vi "ZM_State_heating.vi"(6 "T":u32[](array[numeric])=[300, 180000, 300, 5000, 180000, 3000], 9 "ZB":bool[](array[boolean])=[FALSE, FALSE], 10 "XB":bool[](array[boolean])=[FALSE, FALSE, FALSE, FALSE, FALSE], 11 "Z_In":T4={"Z_Source"=enum."local disabled", "Z_State"=enum."alarm", "ZM_State"=enum."initialization"}) -> (1 "t":u32, 3 "Z_Out":T4={"Z_Source"=enum."local disabled", "Z_State"=enum."alarm", "ZM_State"=enum."initialization"}, 4 "ZM_State_next":u32)   [LabVIEW 2019, in "Heating.lvlib"]
uses:
  Heating.lvlib
  ctl/Y_source.ctl
  ctl/Z_State.ctl
  ctl/ZM_State.ctl
  Trigers/RS.vi
  Timer Delay/Timer.vi
  Userlib.lvlib
panel:
  out "End":bool
  out "Stop":bool
  out "Start":bool
  # "Ki_XB01 contactor on"
  # "Ki_XB02 contactor off"
  # "XB24 local hand on"
  # "heating end"
  # "cooling end"
  # "Ki_ZB01 contactor on reg"
  # "Ki_ZB02 contactor off reg"
  # "T_start_delay"
  # "T_heat_start"
  # "T_stop_delay"
  # "T_set_min"
  # "T_heat_stop"
  # "T_restart_delay"
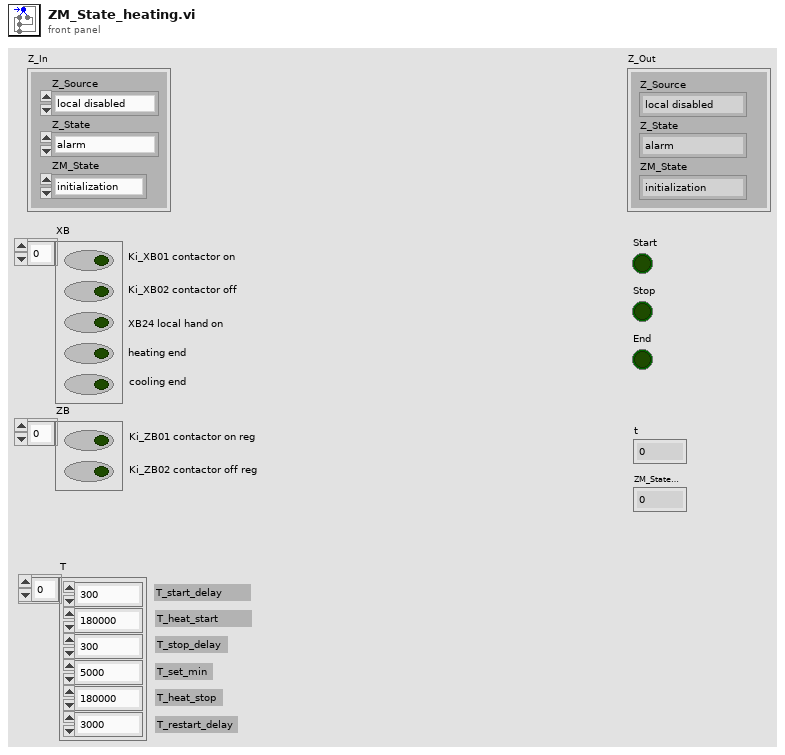
[diagram p1: front panel]
types:
  T1 = typedef "Heating.lvlib/Y_source.ctl" = enum8{"initialize", "local disabled", "local hand", "hand", "auto", "dist"}
  T2 = typedef "Heating.lvlib/Z_State.ctl" = enum8{"initialization", "alarm", "disabled", "not ready", "stop ready", "reserv", "switched off", "reserv2", "switched on", "check", "on min", "decrease out", "on", "increase out", "on max"}
  T3 = typedef "Heating.lvlib/ZM_State.ctl" = enum8{"initialization", "stop", "start_cmd", "contactor_on_cmd", "heating", "on", "stop_cmd", "power_down", "contactor_off_cmd", "cooling", "restart_delay"}
  T4 = cluster{"Z_Source":T1, "Z_State":T2, "ZM_State":T3}
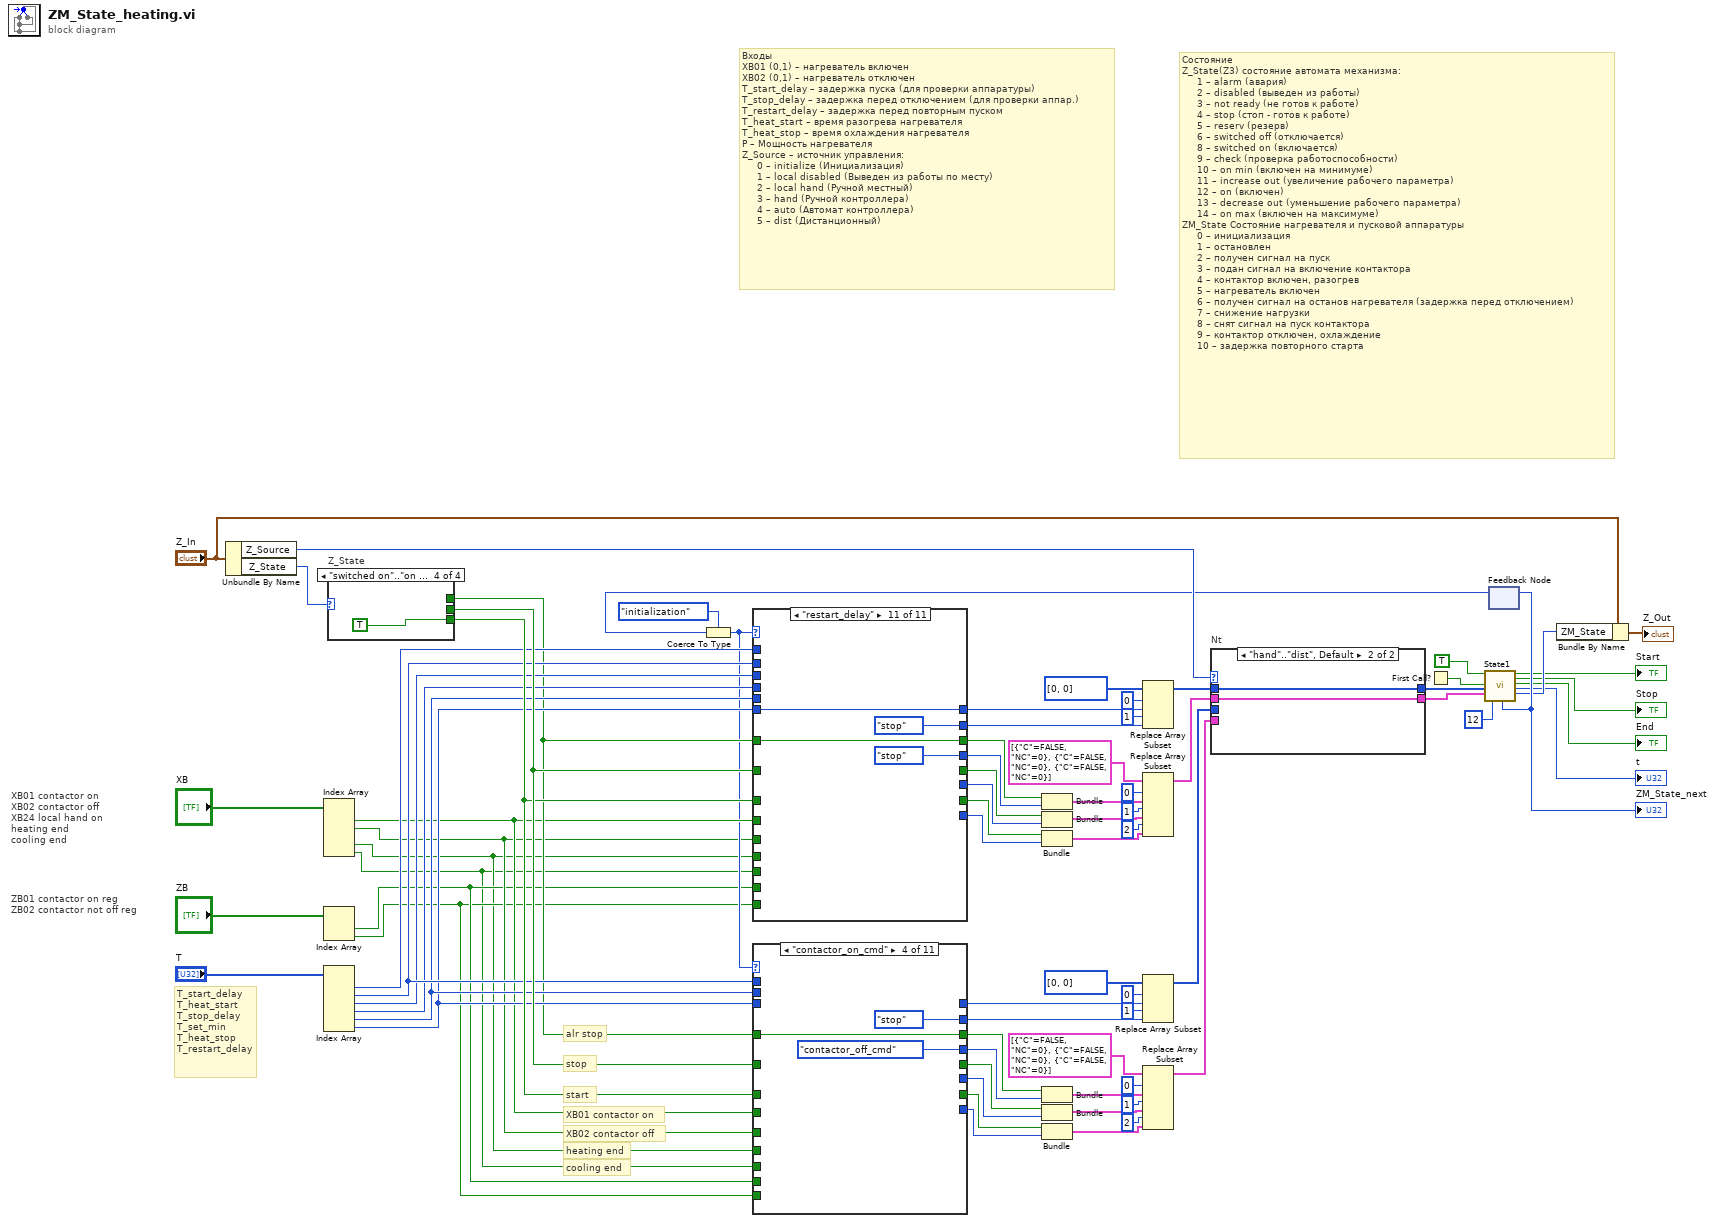
[diagram p0: block diagram]
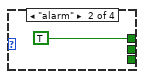
[diagram p3: hidden frame]
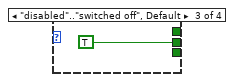
[diagram p4: hidden frame]
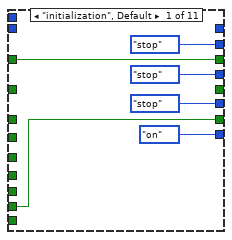
[diagram p5: hidden frame]
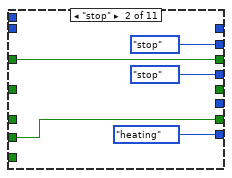
[diagram p6: hidden frame]
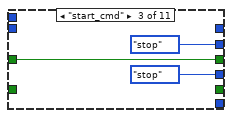
[diagram p7: hidden frame]
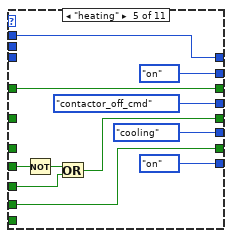
[diagram p8: hidden frame]
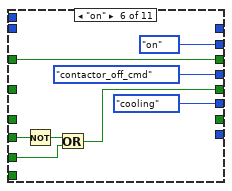
[diagram p9: hidden frame]
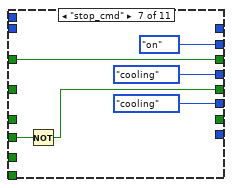
[diagram p10: hidden frame]
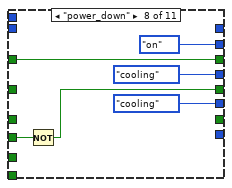
[diagram p11: hidden frame]
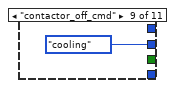
[diagram p12: hidden frame]
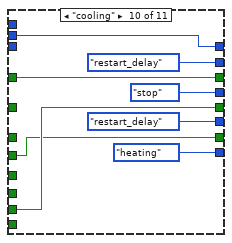
[diagram p13: hidden frame]
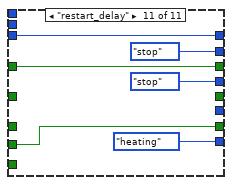
[diagram p14: hidden frame]
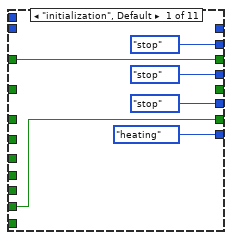
[diagram p15: hidden frame]
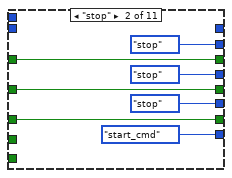
[diagram p16: hidden frame]
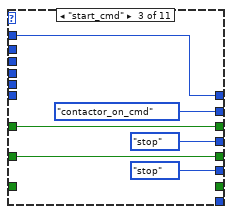
[diagram p17: hidden frame]
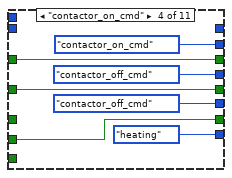
[diagram p18: hidden frame]
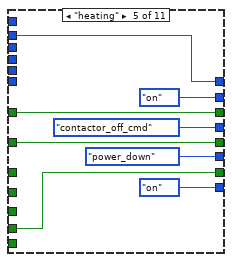
[diagram p19: hidden frame]
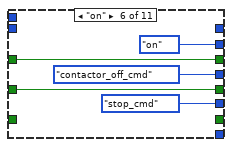
[diagram p20: hidden frame]
diagram:
  # "cooling end"
  # "heating end"
  # "XB02 contactor off"
  # "XB01 contactor on"
  # "Входы\nXB01 (0,1) – нагреватель включен\nXB02 (0,1) – нагреватель отключен\nT_start_delay – задержка пуска (для проверки аппаратуры)\nT_stop_delay – задержка перед отключением (для проверки аппар.)\nT_restart_delay – задержка перед повторным пуском\nT_heat_start – время разогрева нагревателя\nT_heat_stop – время охлаждения нагревателя\nP – Мощность нагревателя\nZ_Source – источник управления:\n     0 – initialize (Инициализация)\n     1 – local disabled (Выведен из работы по месту)\n     2 – local hand (Ручной местный)\n     3 – hand (Ручной контроллера)\n     4 – auto (Автомат контроллера)\n     5 – dist (Дистанционный)"
  # "alr stop"
  # "ZB01 contactor on reg\nZB02 contactor not off reg"
  # "XB01 contactor on\nXB02 contactor off\nXB24 local hand on\nheating end\ncooling end"
  # "T_start_delay\nT_heat_start\nT_stop_delay\nT_set_min\nT_heat_stop\nT_restart_delay"
  # "start"
  # "stop"
  # "Состояние\nZ_State(Z3) состояние автомата механизма:\n     1 – alarm (авария)\n     2 – disabled (выведен из работы)\n     3 – not ready (не готов к работе)\n     4 – stop (стоп - готов к работе)\n     5 – reserv (резерв)\n     6 – switched off (отключается)\n     8 – switched on (включается)\n     9 – check (проверка работоспособности)\n     10 – on min (включен на минимуме)\n     11 – increase out (увеличение рабочего параметра)\n     12 – on (включен)\n     13 – decrease out (уменьшение рабочего параметра)\n     14 – on max (включен на максимуме)\nZM_State Состояние нагревателя и пусковой аппаратуры\n     0 – инициализация\n     1 – остановлен\n     2 – получен сигнал на пуск\n     3 – подан сигнал на включение контактора\n     4 – контактор включен, разогрев\n     5 – нагреватель включен\n     6 – получен сигнал на останов нагревателя (задержка перед отключением)\n     7 – снижение нагрузки\n     8 – снят сигнал на пуск контактора\n     9 – контактор отключен, охлаждение\n     10 – задержка повторного старта"
  n1 = Unbundle By Name("Z_In") -> ("Z_Source"=w63:T1, "Z_State"=w60:T2)
  n2 = Index Array(array="XB") -> (element #1=w65:bool, element #2=w56:bool, element #4=w53:bool, element #5=w52:bool)  [unwired: 5 in, 1 out]
  n3 = Index Array(array="ZB") -> (element #1=w55:bool, element #2=w54:bool)  [unwired: 2 in]
  n4 = Index Array(array="T") -> (element #1=w73:u32, element #2=w72:u32, element #3=w71:u32, element #4=w70:u32, element #5=w69:u32, element #6=w68:u32)  [unwired: 6 in]
  n5 = case "Z_State" shown="\"switched on\"..\"on max\"" w60 {
    tunnel: [_ _ TRUE _] -> w76
    tunnel: [_ _ _ TRUE] -> w75
    tunnel: [_ TRUE _ _] -> w67
    frame "initialization" {
    }
    frame "alarm" {
    }
    frame "disabled".."switched off", Default {
    }
    frame "switched on".."on max" {
    }
  }
  n6 = First Call?() -> (First Call?: T/F=w50:bool)
  n7 = feedback #1() -> (w58:u32)  [unwired: 1 in]
  n8 = Coerce To Type(0:w58, 1:ZM_State."initialization" ("ZM_State")) -> (2:w57:T3)
  n9 = case shown="\"restart_delay\"" w57 {
    tunnel: [_ _ w97 _ w112 _ w122 w125 _ w145 w152] -> w42
    tunnel: [ZM_State."heating" ("ZM_State") ZM_State."start_cmd" ("ZM_State") _ ZM_State."heating" ("ZM_State") ZM_State."on" ("ZM_State") _ ZM_State."on" ("ZM_State") ZM_State."on" ("ZM_State") ZM_State."contactor_on_cmd" ("ZM_State") ZM_State."contactor_on_cmd" ("ZM_State") _] -> w32
    tunnel: [w84 w92 _ w103 w110 _ w123 w129 w141 w144 _] -> w33
    tunnel: [ZM_State."stop" ("ZM_State") ZM_State."stop" ("ZM_State") ZM_State."contactor_on_cmd" ("ZM_State") ZM_State."contactor_on_cmd" ("ZM_State") ZM_State."on" ("ZM_State") ZM_State."on" ("ZM_State") ZM_State."power_down" ("ZM_State") ZM_State."contactor_off_cmd" ("ZM_State") ZM_State."contactor_off_cmd" ("ZM_State") ZM_State."restart_delay" ("ZM_State") ZM_State."stop" ("ZM_State")] -> w41
    tunnel: w76 -> [_ w87 w98 w105 w113 w118 _ _ _ _ _]
    tunnel: w75 -> [_ w92 _ _ _ _ w123 w129 w141 w144 _]
    tunnel: w73 -> [_ _ w97 _ _ _ _ _ _ _ _]
    tunnel: [_ w87 w98 w105 w113 w118 _ _ w135 w143 _] -> w35
    tunnel: [ZM_State."stop" ("ZM_State") ZM_State."stop" ("ZM_State") ZM_State."stop" ("ZM_State") ZM_State."contactor_off_cmd" ("ZM_State") ZM_State."power_down" ("ZM_State") ZM_State."stop_cmd" ("ZM_State") _ _ ZM_State."cooling" ("ZM_State") ZM_State."restart_delay" ("ZM_State") _] -> w34
    tunnel: w65 -> [_ _ _ w103 _ _ _ _ w139 _ _]
    tunnel: w72 -> [_ _ _ _ w112 _ _ _ _ _ _]
    tunnel: w67 -> [w85 w91 w96 w104 w111 w117 w124 w130 w137 w149 w153]
    tunnel: [w85 w91 w96 w104 w111 w117 w124 w130 w136 w149 w153] -> w40
    tunnel: [ZM_State."stop" ("ZM_State") ZM_State."stop" ("ZM_State") ZM_State."stop" ("ZM_State") ZM_State."contactor_off_cmd" ("ZM_State") ZM_State."contactor_off_cmd" ("ZM_State") ZM_State."contactor_off_cmd" ("ZM_State") ZM_State."contactor_off_cmd" ("ZM_State") ZM_State."contactor_off_cmd" ("ZM_State") ZM_State."stop" ("ZM_State") ZM_State."stop" ("ZM_State") ZM_State."stop" ("ZM_State")] -> w39
    tunnel: w71 -> [_ _ _ _ _ _ w122 _ _ _ _]
    tunnel: w70 -> [_ _ _ _ _ _ _ w125 _ _ _]
    tunnel: w56 -> [_ _ _ _ _ _ _ _ w138 _ _]
    tunnel: w69 -> [_ _ _ _ _ _ _ _ _ w145 _]
    tunnel: w68 -> [_ _ _ _ _ _ _ _ _ _ w152]
    tunnel: w55 -> [w84 _ _ _ _ _ _ _ _ _ _]
    tunnel: w54 -> [_ _ _ _ _ _ _ _ _ _ _]
    tunnel: w53 -> [_ _ _ _ w110 _ _ _ _ _ _]
    tunnel: w52 -> [_ _ _ _ _ _ _ _ _ w143 _]
    frame "initialization", Default {
    }
    frame "stop" {
    }
    frame "start_cmd" {
    }
    frame "contactor_on_cmd" {
    }
    frame "heating" {
    }
    frame "on" {
    }
    frame "stop_cmd" {
    }
    frame "power_down" {
    }
    frame "contactor_off_cmd" {
      n10 = Not(x=w139) -> (.not. x?=w140:bool)
      n11 = Or(x=w140, y=w138) -> (x .or. y?=w135:bool)
      n12 = And(x=w137, y=w135) -> (x .and. y?=w136:bool)
    }
    frame "cooling" {
    }
    frame "restart_delay" {
    }
  }
  n13 = case shown="\"contactor_on_cmd\"" w57 {
    tunnel: [_ _ _ _ w181 _ _ _ _ w206 w215] -> w14
    tunnel: [ZM_State."on" ("ZM_State") ZM_State."heating" ("ZM_State") _ _ ZM_State."on" ("ZM_State") _ _ _ _ ZM_State."heating" ("ZM_State") ZM_State."heating" ("ZM_State")] -> w5
    tunnel: [w158 w163 _ _ w171 _ _ _ _ w203 w214] -> w6
    tunnel: [ZM_State."stop" ("ZM_State") ZM_State."stop" ("ZM_State") ZM_State."stop" ("ZM_State") ZM_State."stop" ("ZM_State") ZM_State."on" ("ZM_State") ZM_State."on" ("ZM_State") ZM_State."on" ("ZM_State") ZM_State."on" ("ZM_State") ZM_State."cooling" ("ZM_State") ZM_State."restart_delay" ("ZM_State") ZM_State."stop" ("ZM_State")] -> w13
    tunnel: w76 -> [_ _ _ _ _ _ _ _ _ _ _]
    tunnel: w75 -> [_ _ _ _ _ _ _ _ _ _ _]
    tunnel: [_ _ _ _ w172 w182 w193 w199 _ w204 _] -> w8
    tunnel: [ZM_State."stop" ("ZM_State") _ _ _ ZM_State."cooling" ("ZM_State") ZM_State."cooling" ("ZM_State") ZM_State."cooling" ("ZM_State") ZM_State."cooling" ("ZM_State") _ ZM_State."restart_delay" ("ZM_State") _] -> w7
    tunnel: w65 -> [_ w163 _ _ w174 w184 w194 w200 _ w203 w214]
    tunnel: w72 -> [_ _ _ _ w181 _ _ _ _ _ _]
    tunnel: w67 -> [w159 w164 w167 w170 w180 w189 w195 w201 _ w205 w216]
    tunnel: [w159 w164 w167 w170 w180 w189 w195 w201 _ w205 w216] -> w10
    tunnel: [ZM_State."stop" ("ZM_State") ZM_State."stop" ("ZM_State") ZM_State."stop" ("ZM_State") ZM_State."contactor_off_cmd" ("ZM_State") ZM_State."contactor_off_cmd" ("ZM_State") ZM_State."contactor_off_cmd" ("ZM_State") ZM_State."cooling" ("ZM_State") ZM_State."cooling" ("ZM_State") _ ZM_State."stop" ("ZM_State") ZM_State."stop" ("ZM_State")] -> w9
    tunnel: w56 -> [_ _ _ _ w173 w183 _ _ _ _ _]
    tunnel: w69 -> [_ _ _ _ _ _ _ _ _ w206 _]
    tunnel: w68 -> [_ _ _ _ _ _ _ _ _ _ w215]
    tunnel: w55 -> [w158 _ _ _ _ _ _ _ _ _ _]
    tunnel: w54 -> [_ _ _ _ _ _ _ _ _ _ _]
    tunnel: w53 -> [_ _ _ _ w171 _ _ _ _ _ _]
    tunnel: w52 -> [_ _ _ _ _ _ _ _ _ w204 _]
    frame "initialization", Default {
    }
    frame "stop" {
    }
    frame "start_cmd" {
    }
    frame "contactor_on_cmd" {
    }
    frame "heating" {
      n14 = Not(x=w174) -> (.not. x?=w175:bool)
      n15 = Or(x=w175, y=w173) -> (x .or. y?=w172:bool)
    }
    frame "on" {
      n16 = Not(x=w184) -> (.not. x?=w185:bool)
      n17 = Or(x=w185, y=w183) -> (x .or. y?=w182:bool)
    }
    frame "stop_cmd" {
      n18 = Not(x=w194) -> (.not. x?=w193:bool)
    }
    frame "power_down" {
      n19 = Not(x=w200) -> (.not. x?=w199:bool)
    }
    frame "contactor_off_cmd" {
    }
    frame "cooling" {
    }
    frame "restart_delay" {
    }
  }
  n20 = Bundle(w40, "ZM_State"=w39) -> (w43:cluster{bool, "ZM_State":T3})  [unwired: 1 in]
  n21 = Bundle("XB"=w35, "ZM_State"=w34) -> (w36:cluster{"XB":bool, "ZM_State":T3})  [unwired: 1 in]
  n22 = Bundle("XB"=w33, "ZM_State"=w32) -> (w31:cluster{"XB":bool, "ZM_State":T3})  [unwired: 1 in]
  n23 = Bundle(w10, "ZM_State"=w9) -> (w20:cluster{bool, "ZM_State":T3})  [unwired: 1 in]
  n24 = Bundle("XB"=w8, "ZM_State"=w7) -> (w23:cluster{"XB":bool, "ZM_State":T3})  [unwired: 1 in]
  n25 = Bundle("XB"=w6, "ZM_State"=w5) -> (w24:cluster{"XB":bool, "ZM_State":T3})  [unwired: 1 in]
  n26 = Replace Array Subset(array=u32[] [0, 0] ("appended array"), new element #1=w42, index #1=0 ("index"), new element #2=w41, index #2=1 ("index")) -> (w4:u32[])
  n27 = Replace Array Subset(array=cluster{"C":bool, "NC":u32}[] [{"C"=FALSE, "NC"=0}, {"C"=FALSE, "NC"=0}, {"C"=FALSE, "NC"=0}] ("appended array"), new element #1=w43, index #1=0 ("index"), new element #2=w36, index #2=1 ("index"), new element #3=w31, index #3=2 ("index")) -> (w2:cluster{"C":bool, "NC":u32}[])
  n28 = Replace Array Subset(array=u32[] [0, 0] ("appended array"), new element #1=w14, index #1=0 ("index"), new element #2=w13, index #2=1 ("index")) -> (w12:u32[])
  n29 = Replace Array Subset(array=cluster{"C":bool, "NC":u32}[] [{"C"=FALSE, "NC"=0}, {"C"=FALSE, "NC"=0}, {"C"=FALSE, "NC"=0}] ("appended array"), new element #1=w20, index #1=0 ("index"), new element #2=w23, index #2=1 ("index"), new element #3=w24, index #3=2 ("index")) -> (w11:cluster{"C":bool, "NC":u32}[])
  n30 = case "Nt" shown="\"hand\"..\"dist\", Default" w63 {
    tunnel: w4 -> [_ w220]
    tunnel: w2 -> [_ w219]
    tunnel: [w217 w220] -> w3
    tunnel: [w218 w219] -> w1
    tunnel: w12 -> [w217 _]
    tunnel: w11 -> [w218 _]
    frame "local disabled", "local hand" {
    }
    frame "hand".."dist", Default {
    }
  }
  n31 = call "State1.vi"("Start"=TRUE, "Reset"=w50, "T_table"=w3, "C_table"=w1, "End step"=u32 12) -> ("N next"=w30:u32, "Start"=→"Start":bool, "Stop"=→"Stop":bool, "End"=→"End":bool, "t"=→"t":u32, "N curr"=w29:u32)  [unwired: 9 in]
  "ZM_State_next" <- w30
  n32 = feedback-in #1(w30) -> ()
  n33 = Bundle By Name(cluster="Z_In", "ZM_State"=w29) -> (→"Z_Out":T4)
